vi "Get Font Style.vi"(8 "error in (no error)":errorcluster caption="错误输入（无错误）", 11 "Font 输入":refnum<class "Font.lvclass"> caption="DNL_LabVIEW Object in") -> (0 "error out":errorcluster caption="错误输出", 2 "Style":i32(ring) items=["Regular"=0, "Bold"=1, "Italic"=2, "Underline"=4, "Strikeout"=8], 3 "Font 输出":refnum<class "Font.lvclass"> caption="DNL_LabVIEW Object out")   [LabVIEW 2011, in "Font.lvclass"]
uses:
  Font.lvclass
  Font.lvclass/Font.ctl
  System.Drawing
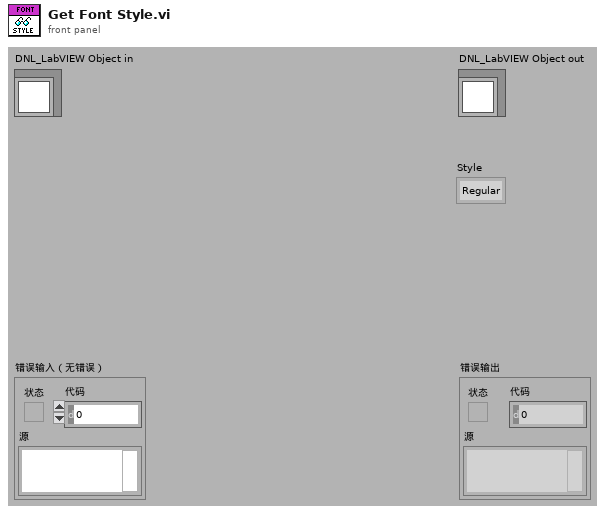
[diagram p1: front panel]
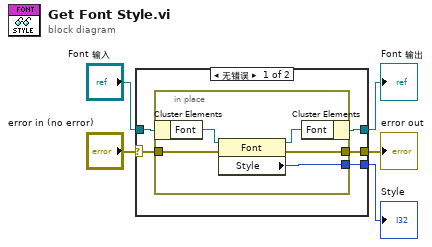
[diagram p0: block diagram]
diagram:
  n1 = case shown="无错误" "error in (no error)" {
    selector: "error in (no error)" -> [w8 w17]
    tunnel: [w7 w17] -> w4
    tunnel: [w9 w16] -> w2
    tunnel: "Font 输入" -> [w10 w16]
    tunnel: [w6 _] -> w1
    frame No Error {
      n2 = in-place {
        in-place-border: w8 -> [w13]
        in-place-border: [w12] -> w7
        in-place-border: [w11] -> w6
        n3 = in-place-cluster #1(w10) -> ("Font"=w15:refnum<k24>)
        n4 = property class="Font"(reference=w15, error in=w13) -> (reference out=w14:refnum<k24>, error out=w12:errorcluster, "Style"=w11:i32)
        n5 = in-place-cluster #1("Font"=w14) -> (w9:refnum<class "Font.lvclass">)
      }
    }
    frame Error {
    }
  }
  "error out" <- w4
  "Font 输出" <- w2
  "Style" <- w1
